vi "Voltage - White Noise - NI (2).vi"() -> ()   [LabVIEW 2022 SP3]
doc: "This example demonstrates how to continuously re-generate analog output data from a buffer in your computer's memory.\n\nRefer to your device documentation for pinouts and hardware capabilities."
uses:
  WhiteNoise.ctl
  <vilib>/Utility/error.llb/DialogType.ctl
  <vilib>/DAQmx/write.llb/DAQmx Write (Analog 1D Wfm NChan NSamp).vi
  <vilib>/DAQmx/create/channels.llb/DAQmx Create Channel (AO-Voltage-Basic).vi
  <vilib>/DAQmx/configure/timing.llb/DAQmx Timing (Sample Clock).vi
  <vilib>/DAQmx/configure/trigger.llb/DAQmx Start Trigger (Digital Edge).vi
  <vilib>/DAQmx/configure/trigger.llb/DAQmx Start Trigger (Time).vi
  <vilib>/DAQmx/configure/trigger.llb/DAQmx Start Trigger (Analog Edge).vi
  <vilib>/measure/maspectr.llb/FFT Spectrum (Mag-Phase) for N Chan.vi
  <vilib>/DAQmx/miscellaneous.llb/DAQmx Fill In Error Info.vi
  <resource>/objmgr/daqmx.rc
  <vilib>/measure/NI_MABase.lvlib
  <vilib>/measure/NI_MAPro.lvlib
panel:
  in  "Reset Averaging":bool
  out "Phase":cluster{"f0":dbl, "df":dbl, "phase":dbl[]}[](graph)
  out "Mag":cluster{"f0":dbl, "df":dbl, "magnitude":dbl[]}[](graph)
  in  "stop":bool
  in  "Iterator":dbl
  in  "Cluster":T2={"Seed"=0.0, "Standard Deviation"=10.0, "Reset"=FALSE} {"Standard Deviation" format="%0.2p"}
  in  "Trigger Type":T3(tab)
  in  "Digital Start Trigger Edge":i32(ring)=10280 caption="Edge" items=["Rising"=10280, "Falling"=10171]
  in  "Digital Start Trigger Source":tag="/Dev1/PFI0" caption="Source"
  in  "Digital Pause Trigger Pause When":i32(ring)=10192 caption="Pause When" items=["High"=10192, "Low"=10214]
  in  "Digital Pause Trigger Source":tag="/Dev1/PFI0" caption="Source"
  in  "Analog Start Trigger Level":dbl caption="Level" format="%0.2f"
  in  "Analog Start Trigger Hysteresis":dbl caption="Hysteresis" format="%.2f"
  in  "Analog Start Trigger Slope":i32(ring)=10280 caption="Slope" items=["Rising"=10280, "Falling"=10171]
  in  "Analog Start Trigger Source":string="APFI0" caption="Source"
  in  "Analog Pause Trigger Source":string="APFI0" caption="Source"
  in  "Analog Pause Trigger Pause When":i32(ring)=10093 caption="Pause When" items=["Above Level"=10093, "Below Level"=10107]
  in  "Analog Pause Trigger Level":dbl caption="Level" format="%.2f"
  in  "When":timestamp
  in  "Select Time\nManually":bool
  in  "Number of Samples":i32=41200
  in  "Stop":bool
  out "Waveform Graph":waveform(dbl)[](graph)=[{"t0"=timestamp(0 s since 1904-01-01), "dt"=0.001, "Y"=[]}]
  in  "Sample Rate":dbl=41200.0
  in  "Sample Clock Source":tag="OnboardClock"
  in  "Max Voltage":dbl=3.5
  in  "Min Voltage":dbl=-3.5
  in  "Physical Channel(s)":tag="Dev1/ao0"
  out "Actual Sample Rate":dbl=1000.0 format="%0.2f"
  # "Channel Settings"
  # "Output"
  # "Timing and\nBuffer Settings"
  # "Waveform Settings"
  # "Trigger Settings"
  # "To enable triggers, select a tab above, and configure the settings.\n\nNot all hardware supports all trigger types. Refer to your device documentation for more information."
  # "This trigger type is not supported in output tasks. \n\nRefer to your device documentation for more information on which triggers are supported."
  # "This trigger type is not supported in output tasks. \n\nRefer to your device documentation for more information on which triggers are supported."
  # "If time is not manually set, task will begin after 10 seconds"
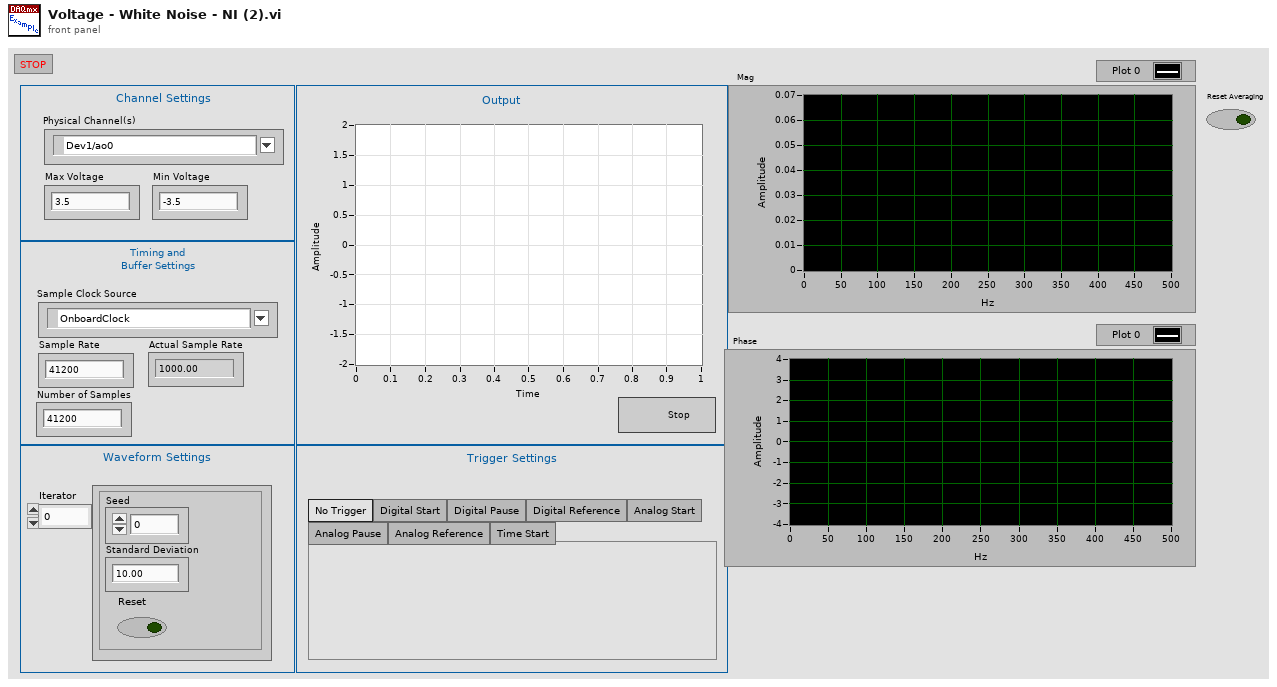
[diagram p1: front panel]
types:
  T1 = typedef "WhiteNoise.ctl" = dbl
  T2 = cluster{"Seed":T1, "Standard Deviation":dbl, "Reset":bool}
  T3 = enum32{"No Trigger", "Digital Start", "Digital Pause", "Digital Reference", "Analog Start", "Analog Pause", "Analog Reference", "Time Start"}
  T4 = typedef "DialogType.ctl" = u16
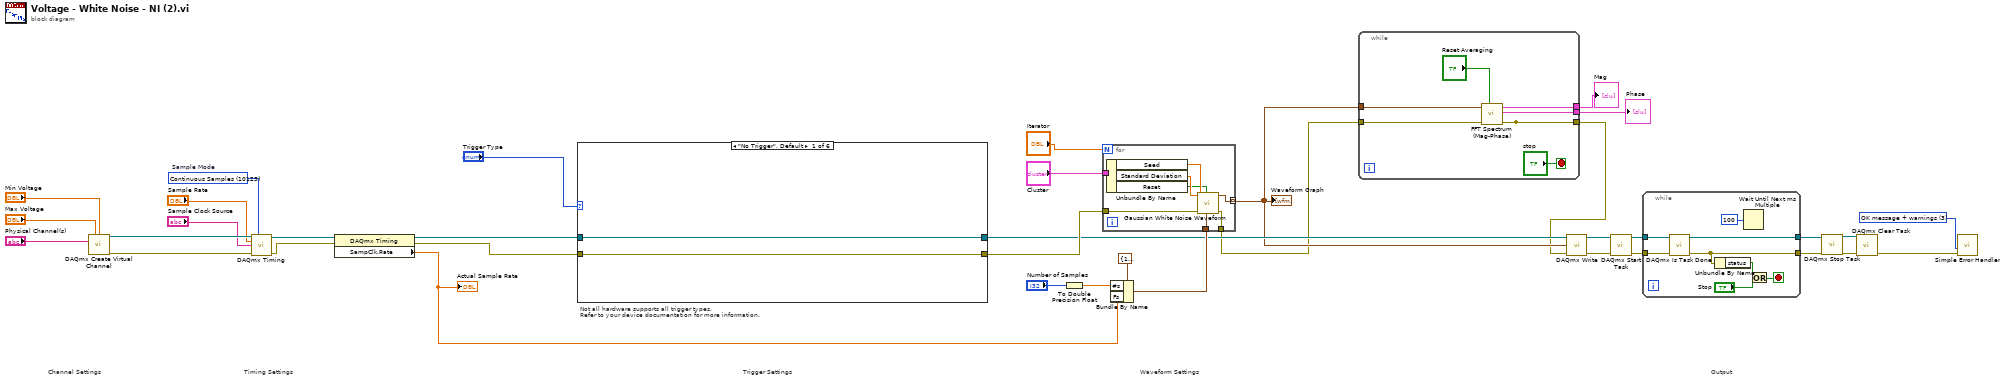
[diagram p0: block diagram]
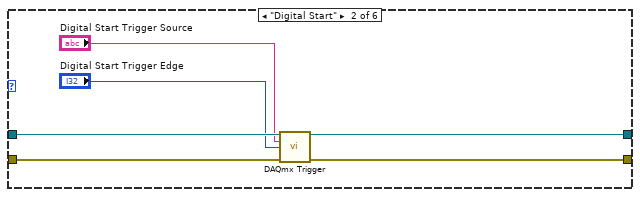
[diagram p2: hidden frame]
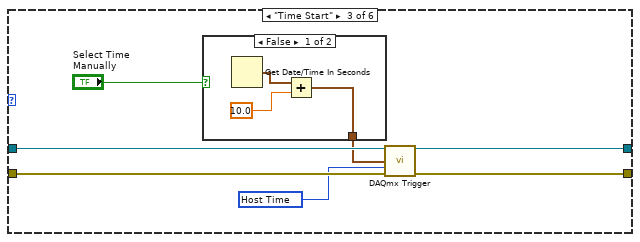
[diagram p3: hidden frame]
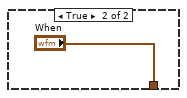
[diagram p4: hidden frame]
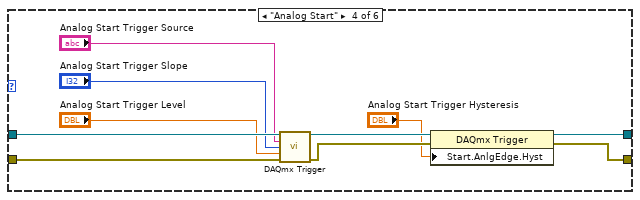
[diagram p5: hidden frame]
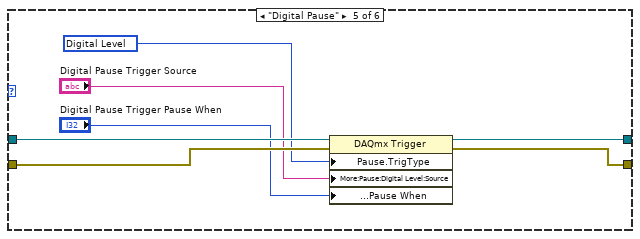
[diagram p6: hidden frame]
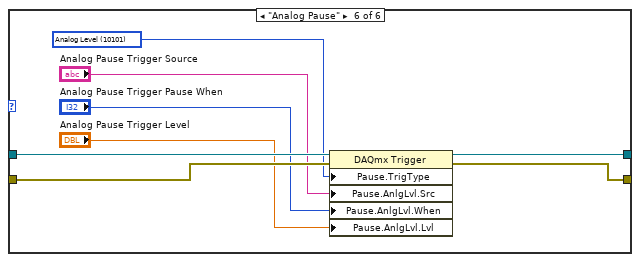
[diagram p7: hidden frame]
diagram:
  w14 = T4 3 items=["no dialog", "OK message", "continue or stop message", "OK message + warnings", "continue/stop + warnings"] ("type of dialog (OK msg:1)")
  w35 = 10123 items=["Finite Samples"=10178, "Continuous Samples"=10123, "Hardware Timed Single Point"=12522]  # Sample Mode
  # "Trigger Settings"
  # "Not all hardware supports all trigger types.\nRefer to your device documentation for more information."
  # "Output"
  # "Waveform Settings"
  # "Timing Settings"
  # "Channel Settings"
  n1 = call-poly <vilib>:"DAQmx Create Virtual Channel.vi"("maximum value"="Max Voltage", "minimum value"="Min Voltage", "physical channels"="Physical Channel(s)") -> ("task out"=w33:refnum<k21>, "error out"=w34:errorcluster)  [unwired: 11 in]
  n2 = call-poly <vilib>:"DAQmx Timing.vi"("task/channels in"=w33, "sample mode"=w35, "rate"="Sample Rate", "source"="Sample Clock Source", "error in"=w34) -> ("task out"=w37:refnum<k21>, "error out"=w36:errorcluster)  [unwired: 9 in]
  n3 = property class="DAQmx Timing"(reference=w37, error in=w36) -> (reference out=w12:refnum<k21>, error out=w11:errorcluster, "SampClk.Rate"=w23:dbl)
  "Actual Sample Rate" <- w23
  n4 = case shown="\"No Trigger\", Default" "Trigger Type" {
    tunnel: w12 -> [w39 w45 w52 w66 w73 w81]
    tunnel: w11 -> [w38 w44 w51 w65 w70 w78]
    tunnel: [w39 w43 w50 w63 w72 w80] -> w9
    tunnel: [w38 w42 w49 w62 w71 w79] -> w10
    frame "No Trigger", Default {
    }
    frame "Digital Start" {
      n5 = call-poly <vilib>:"DAQmx Trigger.vi"("task/channels in"=w45, "source"="Digital Start Trigger Source", "edge"="Digital Start Trigger Edge", "error in"=w44) -> ("task out"=w43:refnum<k21>, "error out"=w42:errorcluster)  [unwired: 10 in]
    }
    frame "Time Start" {
      w48 = 16126 items=["Host Time"=16126, "I/O Device Time"=16127] ("timescale")
      n6 = case shown="False" "Select Time\nManually" {
        tunnel: [w54 "When"] -> w46
        frame False {
          n7 = Get Date/Time In Seconds() -> (seconds since 1Jan1904=w55:timestamp)
          n8 = Add(x=w55, y=10.0) -> (x+y=w54:timestamp)
        }
        frame True {
        }
      }
      n9 = call-poly <vilib>:"DAQmx Trigger.vi"("task/channels in"=w52, "when"=w46, "timescale"=w48, "error in"=w51) -> ("task out"=w50:refnum<k21>, "error out"=w49:errorcluster)  [unwired: 10 in]
    }
    frame "Analog Start" {
      n10 = call-poly <vilib>:"DAQmx Trigger.vi"("task/channels in"=w66, "source"="Analog Start Trigger Source", "slope"="Analog Start Trigger Slope", "level"="Analog Start Trigger Level", "error in"=w65) -> ("task out"=w61:refnum<k21>, "error out"=w60:errorcluster)  [unwired: 9 in]
      n11 = property class="DAQmx Trigger"(reference=w61, error in=w60, "Start.AnlgEdge.Hyst"="Analog Start Trigger Hysteresis") -> (reference out=w63:refnum<k21>, error out=w62:errorcluster)
    }
    frame "Digital Pause" {
      w69 = 10152 items=["Analog Level"=10101, "Analog Window"=10103, "Digital Level"=10152, "Digital Pattern"=10398, "None"=10230] ("Pause.TrigType")
      n12 = property class="DAQmx Trigger"(reference=w73, error in=w70, "Pause.TrigType"=w69, "More:Pause:Digital Level:Source"="Digital Pause Trigger Source", "More:Pause:Digital Level:Pause When"="Digital Pause Trigger Pause When") -> (reference out=w72:refnum<k21>, error out=w71:errorcluster)
    }
    frame "Analog Pause" {
      w77 = 10101 items=["Analog Level"=10101, "Analog Window"=10103, "Digital Level"=10152, "Digital Pattern"=10398, "None"=10230] ("Pause.TrigType")
      n13 = property class="DAQmx Trigger"(reference=w81, error in=w78, "Pause.TrigType"=w77, "Pause.AnlgLvl.Src"="Analog Pause Trigger Source", "Pause.AnlgLvl.When"="Analog Pause Trigger Pause When", "Pause.AnlgLvl.Lvl"="Analog Pause Trigger Level") -> (reference out=w80:refnum<k21>, error out=w79:errorcluster)
    }
  }
  n14 = To Double Precision Float(number="Number of Samples") -> (double precision float=w20:dbl)
  n15 = Bundle By Name(cluster=cluster{"Fs":dbl, "#s":dbl} {"Fs"=1000.0, "#s"=1000.0} ("sampling info"), "#s"=w20, "Fs"=w23) -> (w22:cluster{"Fs":dbl, "#s":dbl})
  n16 = for {
    N: "Iterator" -> [_]
    tunnel: w10 -> [w89]
    tunnel: w22 -> [w88]
    tunnel: [w87] -> w2
    tunnel: "Cluster" -> [w86]
    tunnel: [w85] -> w3 mode=indexing
    n17 = Unbundle By Name(w86) -> ("Seed"=w84:T1, "Standard Deviation"=w83:dbl, "Reset"=w82:bool)
    n18 = call <vilib>:"Gaussian White Noise Waveform.vi"("sampling info"=w88, "reset signal"=w82, "error in (no error)"=w89, "seed"=w84, "standard deviation"=w83) -> ("error out"=w87:errorcluster, "signal out"=w85:waveform(dbl))  [unwired: 5 in]
  }
  "Waveform Graph" <- w3
  n19 = while {
    tunnel: [w95] -> w6
    tunnel: [w94] -> w5
    tunnel: [w91] -> _
    tunnel: w2 -> [w93]
    tunnel: w3 -> [w92]
    tunnel: [w91] -> w1
    stop <- "stop" stop-if-true
    n20 = call-poly <vilib>:"FFT Spectrum (Mag-Phase).vi"("restart averaging (F)"="Reset Averaging", "error in (no error)"=w93, "time signals"=w92) -> ("error out"=w91:errorcluster, "phases"=w95:cluster{"f0":dbl, "df":dbl, "phase":dbl[]}[], "magnitudes"=w94:cluster{"f0":dbl, "df":dbl, "magnitude":dbl[]}[])  [unwired: 4 in, 2 out]
  }
  "Phase" <- w6
  "Mag" <- w5
  n21 = call-poly <vilib>:"DAQmx Write.vi"("task/channels in"=w9, "data"=w3, "error in"=w1) -> ("task out"=w21:refnum<k21>, "error out"=w4:errorcluster)  [unwired: 10 in, 1 out]
  n22 = call <vilib>:"DAQmx Start Task.vi"("task/channels in"=w21, "error in"=w4) -> ("task out"=w32:refnum<k21>, "error out"=w31:errorcluster)  [unwired: 12 in]
  n23 = while {
    tunnel: w32 -> [w104]
    tunnel: w31 -> [w103]
    tunnel: [w100] -> w15
    tunnel: [w101] -> w16
    stop <- w102 stop-if-true
    n24 = call <vilib>:"DAQmx Is Task Done.vi"("task/channels in"=w104, "error in"=w103) -> ("task out"=w101:refnum<k21>, "error out"=w100:errorcluster)  [unwired: 11 in, 1 out]
    n25 = Unbundle By Name(w100) -> ("status"=w99:bool)
    n26 = Wait Until Next ms Multiple(millisecond multiple=u32 100) -> ()  [unwired: 1 out]
    n27 = Or(x=w99, y="Stop") -> (x .or. y?=w102:bool)
  }
  n28 = call <vilib>:"DAQmx Stop Task.vi"("task/channels in"=w16, "error in"=w15) -> ("task out"=w18:refnum<k21>, "error out"=w17:errorcluster)  [unwired: 12 in]
  n29 = call <vilib>:"DAQmx Clear Task.vi"("task in"=w18, "error in"=w17) -> ("error out"=w30:errorcluster)  [unwired: 13 in]
  n30 = call <vilib>:"Simple Error Handler.vi"("type of dialog (OK msg:1)"=w14, "error in (no error)"=w30) -> ()  [unwired: 3 in, 5 out]
